vi "16CH Denkovi Manager.vi"(7 "Action":T2=enum."Init", 8 "error in (no error)":errorcluster, 9 "Relay #":i8 min=1 max=8, 10 "Relays In":bool[](array[boolean])=[FALSE, FALSE, FALSE, FALSE, FALSE, FALSE, FALSE, FALSE, FALSE, FALSE, FALSE, FALSE, FALSE, FALSE, FALSE, FALSE]) -> (0 "error out":errorcluster, 2 "Relays Out":bool[](array[boolean]), 4 "Connected":bool)   [LabVIEW 2020]
uses:
  16CH Denkovi Mngr.ctl
  <vilib>/Instr/_visa.llb/VISA Find Search Mode.ctl
  Hardware Globals.vi
panel:
  out "find list 2":string[](array[string])
  out "find list":string[](array[string])
  out "Device Description":string
  out "Pin States":T1
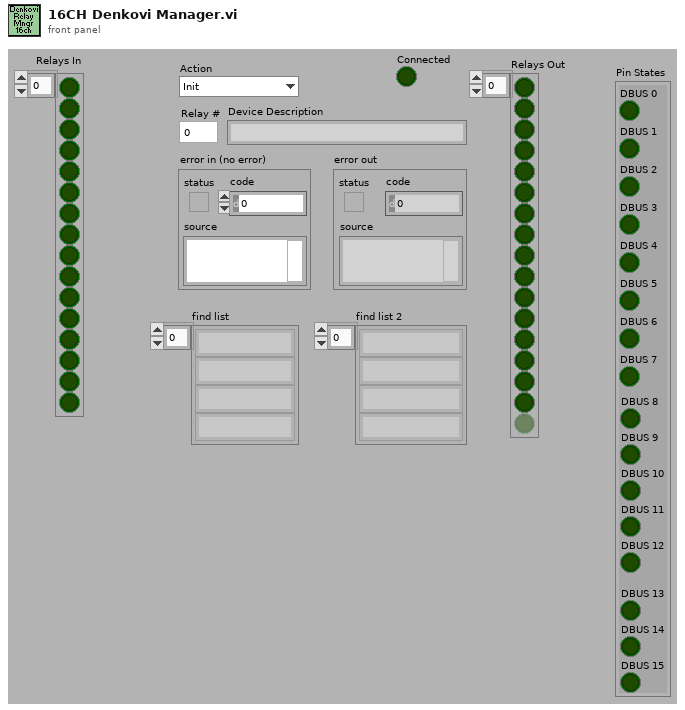
[diagram p1: front panel]
types:
  T1 = cluster{"DBUS 0":bool, "DBUS 1":bool, "DBUS 2":bool, "DBUS 3":bool, "DBUS 4":bool, "DBUS 5":bool, "DBUS 6":bool, "DBUS 7":bool, "DBUS 8":bool, "DBUS 9":bool, "DBUS 10":bool, "DBUS 11":bool, "DBUS 12":bool, "DBUS 13":bool, "DBUS 14":bool, "DBUS 15":bool}
  T2 = typedef "16CH Denkovi Mngr.ctl" = enum16{"Search", "Init", "Set Peristaltic", "Set Pressure", "Set Vacuum", "Pres Vent&Close", "Vac Vent&Close", "Pres ON", "Vac ON", "Set All Relays", "Set One Relay", "Read Relays", "Close"}
  T3 = typedef "VISA Find Search Mode.ctl" = u32
  T4 = cluster{"Boolean array[0]":bool, "Boolean array[1]":bool, "Boolean array[2]":bool, "Boolean array[3]":bool, "Boolean array[4]":bool, "Boolean array[5]":bool, "Boolean array[6]":bool, "Boolean array[7]":bool, "Boolean array[8]":bool, "Boolean array[9]":bool, "Boolean array[10]":bool, "Boolean array[11]":bool, "Boolean array[12]":bool, "Boolean array[13]":bool, "Boolean array[14]":bool, "Boolean array[15]":bool}
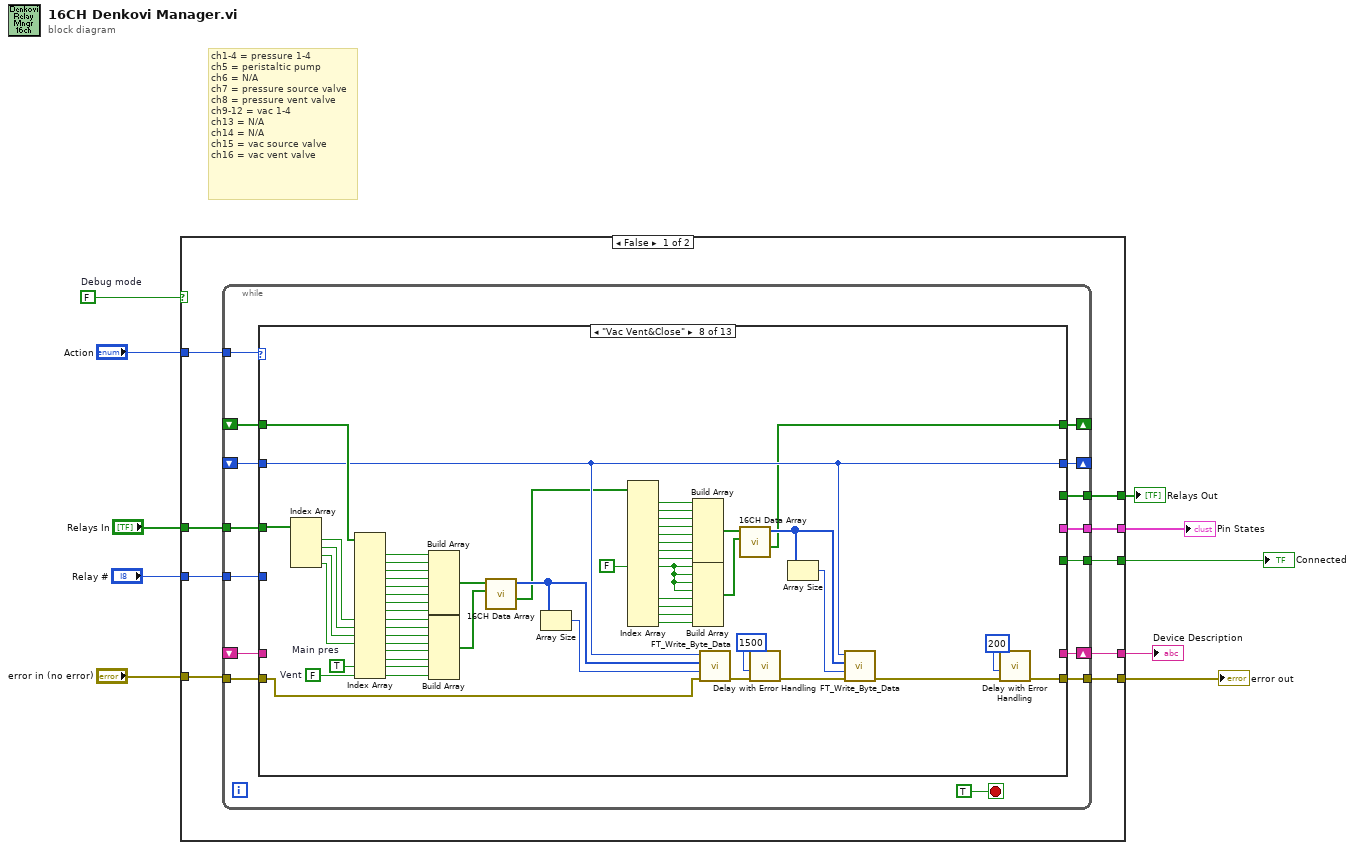
[diagram p0: block diagram]
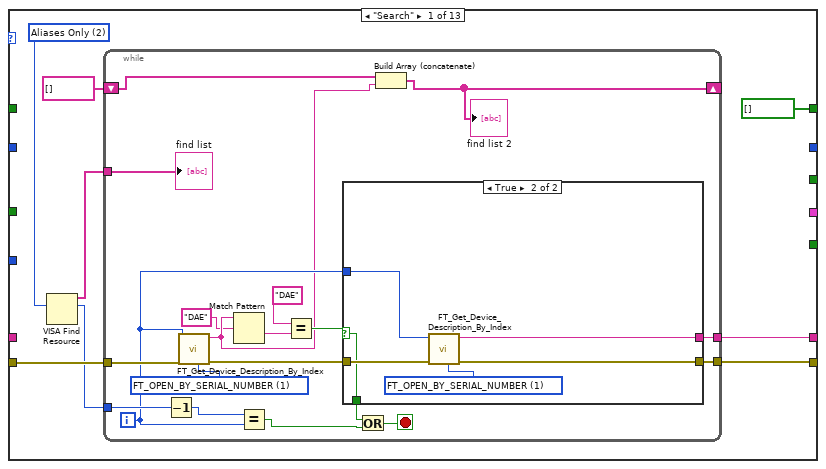
[diagram p2: hidden frame]
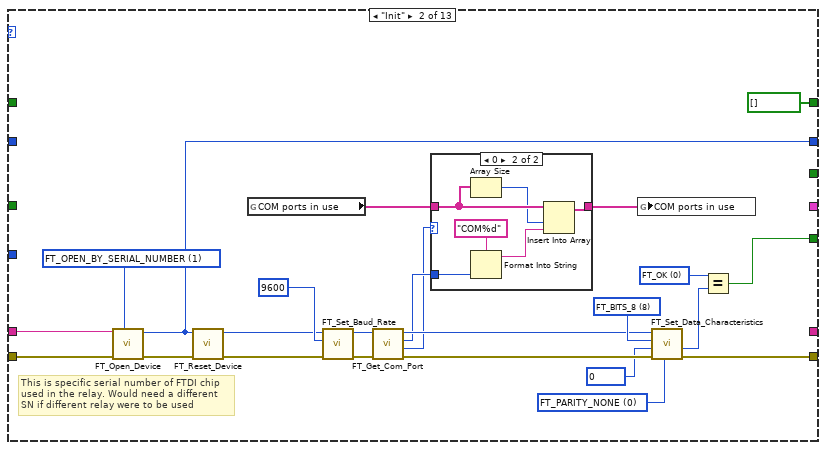
[diagram p4: hidden frame]
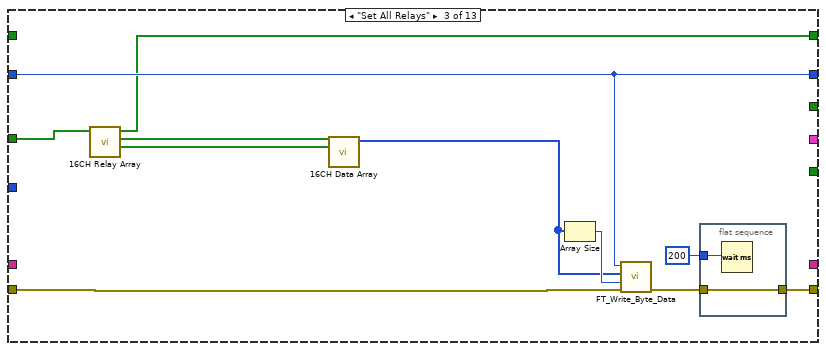
[diagram p6: hidden frame]
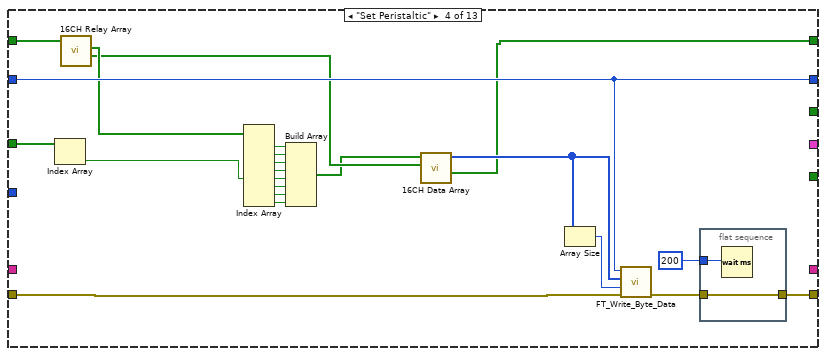
[diagram p7: hidden frame]
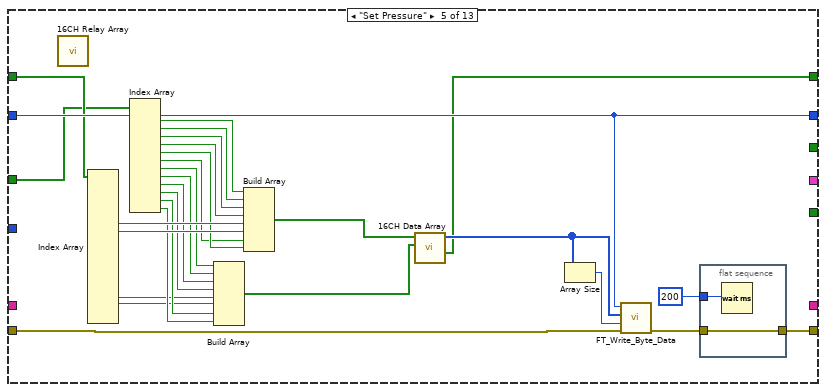
[diagram p8: hidden frame]
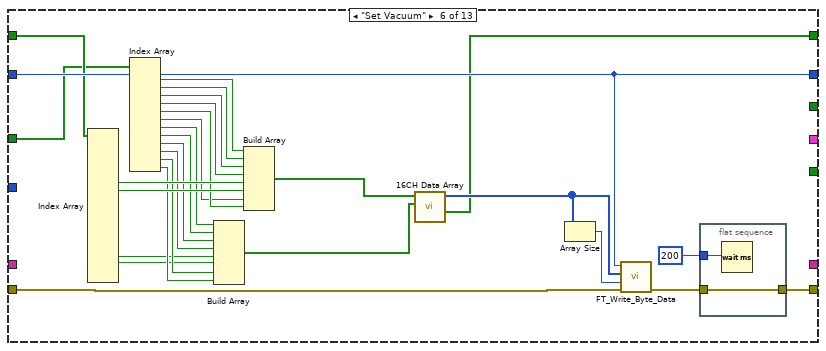
[diagram p9: hidden frame]
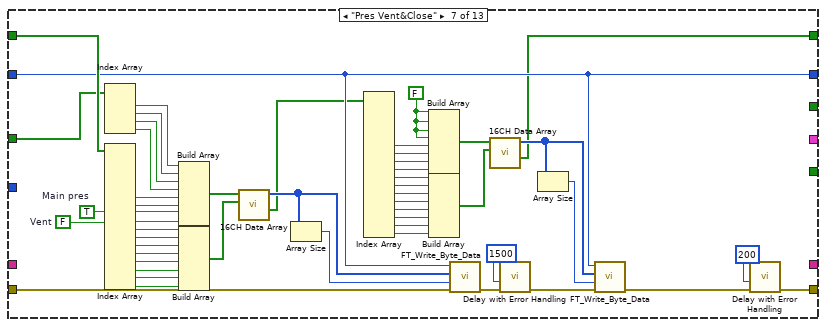
[diagram p10: hidden frame]
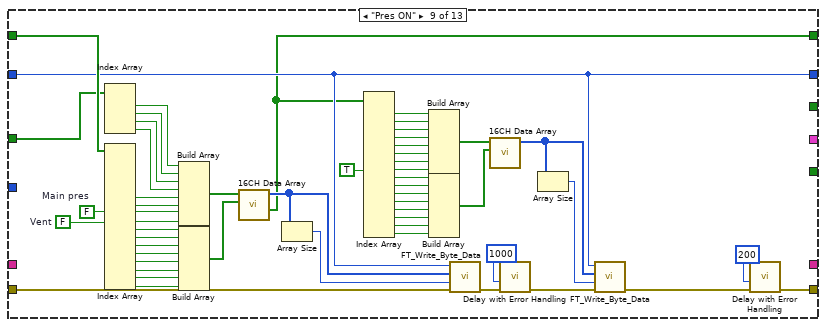
[diagram p11: hidden frame]
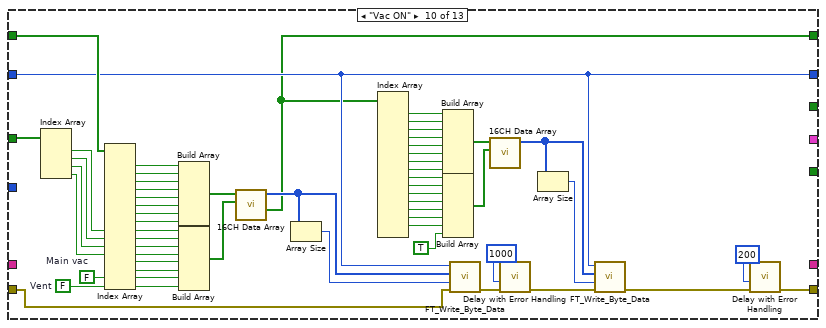
[diagram p12: hidden frame]
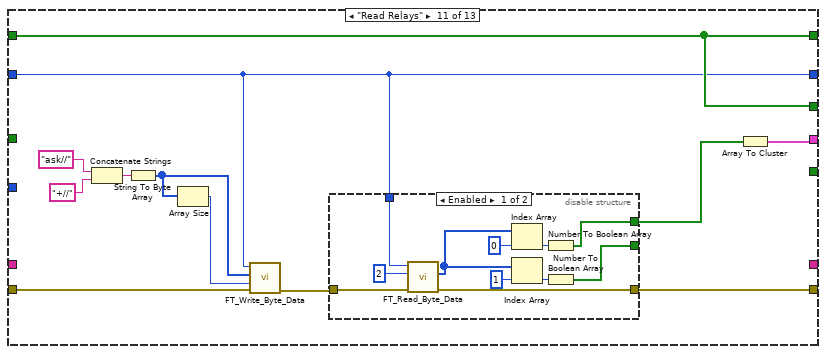
[diagram p13: hidden frame]
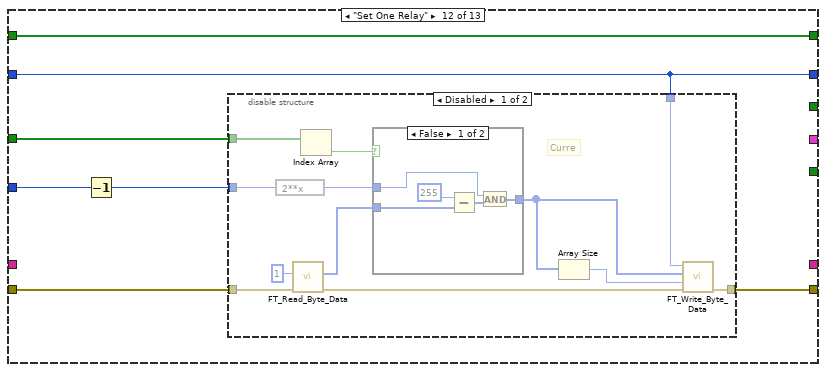
[diagram p15: hidden frame]
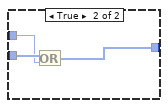
[diagram p16: hidden frame]
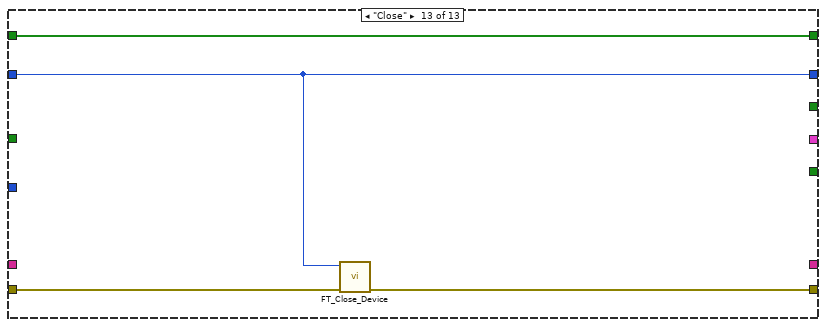
[diagram p18: hidden frame]
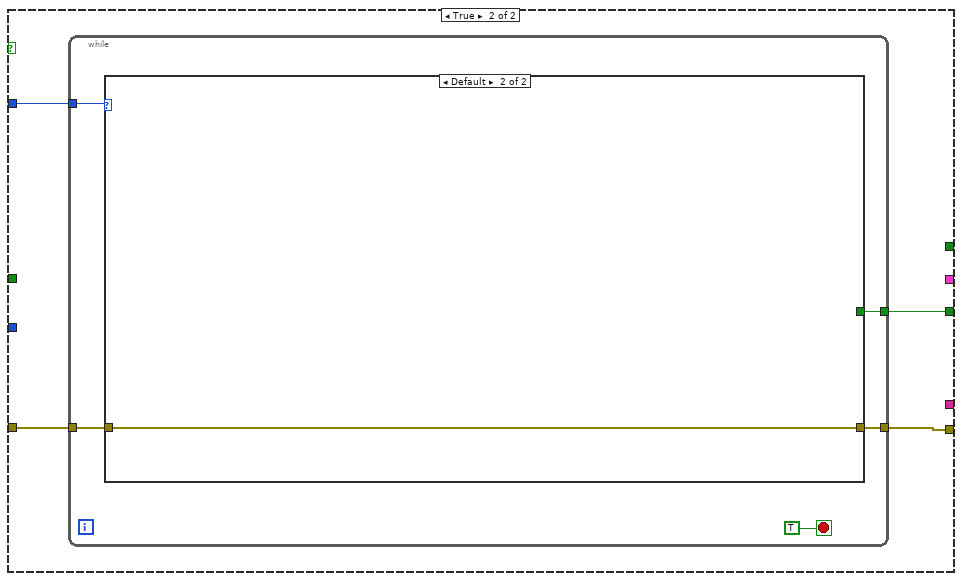
[diagram p19: hidden frame]
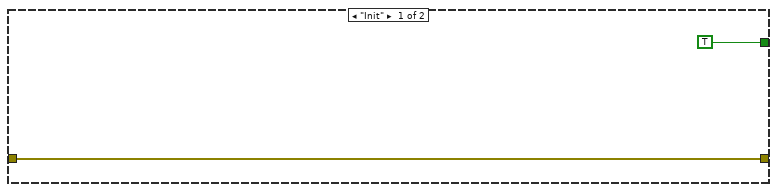
[diagram p20: hidden frame]
diagram:
  w3 = FALSE  # Debug mode
  # "ch1-4 = pressure 1-4\nch5 = peristaltic pump\nch6 = N/A\nch7 = pressure source valve\nch8 = pressure vent valve\nch9-12 = vac 1-4\nch13 = N/A\nch14 = N/A\nch15 = vac source valve\nch16 = vac vent valve"
  n1 = case shown="False" w3 {
    tunnel: [w19 w454] -> w10
    tunnel: "error in (no error)" -> [w18 w453]
    tunnel: "Action" -> [w17 w452]
    tunnel: [w16 w451] -> w7
    tunnel: "Relays In" -> [w15 _]
    tunnel: [w14 _] -> w1
    tunnel: "Relay #" -> [w13 _]
    tunnel: [w12 _] -> w4
    tunnel: [w11 _] -> w2
    frame False {
      n2 = while {
        tunnel: w18 -> [w32]
        tunnel: [w31] -> w19
        tunnel: w17 -> [w33]
        tunnel: [w30] -> w16
        shift-right: [w29] -> _
        shift-left: _ -> [w28]
        tunnel: w15 -> [w27]
        tunnel: [w20] -> w14
        tunnel: w13 -> [w26]
        tunnel: [w25] -> w12
        shift-right: [w24] -> _
        shift-left: _ -> [w23]
        shift-right: [w22] -> w11
        shift-left: _ -> [w21]
        stop <- TRUE stop-if-true
        n3 = case shown="\"Vac Vent&Close\"" w33 {
          tunnel: w32 -> [w42 w82 w106 w128 w158 w188 w242 w291 w342 w393 w404 w422 w450]
          tunnel: [w39 w86 w107 w130 w160 w190 w225 w281 w326 w383 w407 w425 w449] -> w31
          tunnel: [_ w92 _ _ _ _ _ _ _ _ _ _ _] -> w30
          tunnel: [_ w73 w109 w132 w162 w192 w222 w278 w324 w380 w399 w424 w448] -> w29
          tunnel: w28 -> [_ _ w109 w132 w162 w192 w222 w278 w324 w380 w399 w424 w448]
          tunnel: w27 -> [_ _ w104 w124 w154 w184 w238 w256 w338 w359 _ w426 _]
          tunnel: w26 -> [_ _ _ _ _ _ _ _ _ _ _ w423 _]
          tunnel: [_ _ _ _ _ _ _ _ _ _ w406 _ _] -> w25
          tunnel: [bool[] [] ("Relays In") bool[] [] ("Relays In") w100 w113 w136 w166 w196 w245 w299 w350 w406 w420 w447] -> w24
          tunnel: w23 -> [_ _ _ w120 w157 w187 w241 w290 w341 w392 w406 w420 w447]
          tunnel: [w36 _ _ _ _ _ _ _ _ _ _ _ _] -> w22
          tunnel: w21 -> [_ w72 _ _ _ _ _ _ _ _ _ _ _]
          tunnel: [_ _ _ _ _ _ _ _ _ _ w405 _ _] -> w20
          frame "Search" {
            w41 = T3 2 items=["Canonical Names Only"=0, "Aliases Only"=2, "Include Matching Aliases"=3, "Include All Aliases"=4] ("Search Mode")
            n4 = VISA Find Resource(10:w41) -> (2:w40:u32, 3:w37:string[])  [unwired: 2 in, 1 out]
            n5 = while {
              tunnel: w42 -> [w61]
              tunnel: w40 -> [w58]
              tunnel: [w55] -> w39
              tunnel: w37 -> [w53]
              tunnel: [w52] -> w36
              shift-right: [w50] -> _
              shift-left: string[] [] -> [w51]
              i -> [w54]
              stop <- w45 stop-if-true
              w49 = u32 1 items=["FT_OPEN_BY_SERIAL_NUMBER"=1, "FT_OPEN_BY_DESCRIPTION"=2, "FT_OPEN_BY_LOCATION"=4] ("Flags")
              n6 = Decrement(x=w58) -> (x-1=w57:u32)
              n7 = call "FT_Get_Device_Description_By_Index.vi"("Flags"=w49, "error in (no error)"=w61, "Device Index"=w54) -> ("error out"=w59:errorcluster, "Device Description"=w44:string)  [unwired: 6 in, 1 out]
              n8 = Match Pattern(string=w44, regular expression="DAE" ("string")) -> (match substring=w48:string)  [unwired: 1 in, 3 out]
              n9 = Equal?(x=w57, y=w54) -> (x = y?=w47:bool)
              n10 = Equal?(x="DAE", y=w48) -> (x = y?=w56:bool)
              n11 = case shown="True" w56 {
                selector: w56 -> [_ w64]
                tunnel: w59 -> [w62 w68]
                tunnel: [w62 w66] -> w55
                tunnel: w54 -> [_ w67]
                tunnel: [_ w65] -> w52
                tunnel: [_ w64] -> w46
                frame False {
                }
                frame True {
                  w63 = u32 1 items=["FT_OPEN_BY_SERIAL_NUMBER"=1, "FT_OPEN_BY_DESCRIPTION"=2, "FT_OPEN_BY_LOCATION"=4] ("Flags")
                  n12 = call "FT_Get_Device_Description_By_Index.vi"("Flags"=w63, "error in (no error)"=w68, "Device Index"=w67) -> ("error out"=w66:errorcluster, "Device Description"=w65:string)  [unwired: 6 in, 1 out]
                }
              }
              n13 = Or(x=w46, y=w47) -> (x .or. y?=w45:bool)
              n14 = Build Array (concatenate)(w51, w44) -> (w50:string[])
              "find list 2" <- w50
              "find list" <- w53
            }
          }
          frame "Init" {
            w71 = u8 0 items=["FT_STOP_BITS_1"=1, "FT_STOP_BITS_2"=2] ("Stop Bits")
            w83 = u32 1 items=["FT_OPEN_BY_SERIAL_NUMBER"=1, "FT_OPEN_BY_DESCRIPTION"=2, "FT_OPEN_BY_LOCATION"=4] ("Flags")
            w89 = u8 0 items=["FT_PARITY_NONE", "FT_PARITY_ODD", "FT_PARITY_EVEN", "FT_PARITY_MARK", "FT_PARITY_SPACE"] ("Parity")
            w88 = u8 8 items=["FT_BITS_7"=7, "FT_BITS_8"=8] ("Word Length")
            w91 = u32 0 items=["FT_OK", "FT_INVALID_HANDLE", "FT_DEVICE_NOT_FOUND", "FT_DEVICE_NOT_OPENED", "FT_IO_ERROR", "FT_INSUFFICIENT_RESOURCES", "FT_INVALID_PARAMETER", "FT_INVALID_BAUD_RATE", "FT_DEVICE_NOT_OPENED_FOR_ERASE", "FT_DEVICE_NOT_OPENED_FOR_WRITE", "FT_FAILED_TO_WRITE_DEVICE", "FT_EEPROM_READ_FAILED", "FT_EEPROM_WRITE_FAILED", "FT_EEPROM_ERASE_FAILED", "FT_EEPROM_NOT_PRESENT", "FT_EEPROM_NOT_PROGRAMMED", "FT_INVALID_ARGS", "FT_NOT_SUPPORTED", "FT_OTHER_ERROR"] ("FT_Status")
            # "This is specific serial number of FTDI chip\nused in the relay. Would need a different\nSN if different relay were to be used"
            n15 = call "FT_Open_Device.vi"("Flags"=w83, "error in (no error)"=w82, "Device Description"=w72) -> ("error out"=w85:errorcluster, "Handle"=w73:u64)  [unwired: 6 in, 1 out]
            n16 = call "FT_Reset_Device.vi"("error in (no error)"=w85, "Handle In"=w73) -> ("error out"=w69:errorcluster, "Handle Out"=w70:u64)  [unwired: 7 in, 1 out]
            n17 = global read "Hardware Globals.vi" "COM ports in use"() -> (w76:string[])
            n18 = call "FT_Set_Baud_Rate.vi"("error in (no error)"=w69, "Baud Rate"=9600, "Handle  In"=w70) -> ("error out"=w81:errorcluster, "Handle Out"=w80:u64)  [unwired: 6 in, 1 out]
            n19 = call "FT_Get_Com_Port.vi"("error in (no error)"=w81, "Handle In"=w80) -> ("error out"=w78:errorcluster, "FT_Status"=w74:u32, "ComPortNumber"=w77:i32, "Handle Out"=w79:u64)  [unwired: 6 in]
            n20 = case shown="0" w74 {
              tunnel: w77 -> [_ w99]
              tunnel: w76 -> [w93 w97]
              tunnel: [w93 w94] -> w75
              frame Default {
              }
              frame 0 {
                n21 = Array Size(array=w97) -> (size(s)=w96:i32)
                n22 = Format Into String(format string="COM%d", w99) -> (resulting string=w95:string)  [unwired: 2 in, 1 out]
                n23 = Insert Into Array(array=w97, index=w96, new element=w95) -> (w94:string[])
              }
            }
            n24 = global write "Hardware Globals.vi" "COM ports in use"(w75) -> ()
            n25 = call "FT_Set_Data_Characteristics.vi"("Parity"=w89, "error in"=w78, "Stop Bits"=w71, "Word Length"=w88, "Handle In"=w79) -> ("error out"=w86:errorcluster, "FT_Status"=w87:u32)  [unwired: 4 in, 1 out]
            n26 = Equal?(x=w91, y=w87) -> (x = y?=w92:bool)
          }
          frame "Set All Relays" {
            n27 = call "16CH Relay Array.vi"("Relays In"=w104) -> ("Relays 9-16"=w102:bool[], "Relays 1-8"=w103:bool[], "Relays 1-16"=w100:bool[])  [unwired: 8 in]
            n28 = call "16CH Data Array.vi"("Relays 9-16"=w102, "Relays 1-8"=w103) -> ("unsigned byte array"=w105:u8[])  [unwired: 8 in, 1 out]
            n29 = Array Size(array=w105) -> (size(s)=w110:i32)
            n30 = call "FT_Write_Byte_Data.vi"("error in (no error)"=w106, "Bytes To Write"=w110, "Buffer"=w105, "Handle"=w109) -> ("error out"=w108:errorcluster)  [unwired: 4 in, 3 out]
            n31 = flat-sequence {
              tunnel: w108 -> [w112]
              tunnel: [w112] -> w107
              tunnel: u32 200 ("Delay (ms)") -> [w111]
              frame #0 {
                n32 = Wait (ms)(milliseconds to wait=w111) -> ()  [unwired: 1 out]
              }
            }
          }
          frame "Set Peristaltic" {
            n33 = Index Array(array=w124) -> (element=w114:bool)  [unwired: 1 in]
            n34 = call "16CH Relay Array.vi"("Relays In"=w120) -> ("Relays 9-16"=w118:bool[], "Relays 1-8"=w119:bool[])  [unwired: 8 in, 1 out]
            n35 = Index Array(array=w119) -> (element #1=w127:bool, element #2=w126:bool, element #3=w125:bool, element #4=w115:bool, element #6=w121:bool, element #7=w122:bool, element #8=w123:bool)  [unwired: 8 in, 1 out]
            n36 = Build Array(w127, w126, w125, w115, w114, w121, w122, w123) -> (w117:bool[])
            n37 = call "16CH Data Array.vi"("Relays 9-16"=w118, "Relays 1-8"=w117) -> ("Relays 1-16"=w113:bool[], "unsigned byte array"=w116:u8[])  [unwired: 8 in]
            n38 = Array Size(array=w116) -> (size(s)=w133:i32)
            n39 = call "FT_Write_Byte_Data.vi"("error in (no error)"=w128, "Bytes To Write"=w133, "Buffer"=w116, "Handle"=w132) -> ("error out"=w131:errorcluster)  [unwired: 4 in, 3 out]
            n40 = flat-sequence {
              tunnel: w131 -> [w135]
              tunnel: [w135] -> w130
              tunnel: u32 200 ("Delay (ms)") -> [w134]
              frame #0 {
                n41 = Wait (ms)(milliseconds to wait=w134) -> ()  [unwired: 1 out]
              }
            }
          }
          frame "Set Pressure" {
            n42 = call "16CH Relay Array.vi"() -> ()  [unwired: 9 in, 3 out]
            n43 = Index Array(array=w157) -> (element #5=w155:bool, element #6=w156:bool, element #14=w140:bool, element #15=w141:bool)  [unwired: 17 in, 13 out]
            n44 = Index Array(array=w154) -> (element #1=w153:bool, element #2=w152:bool, element #3=w151:bool, element #4=w150:bool, element #5=w149:bool, element #6=w148:bool, element #7=w142:bool, element #8=w143:bool, element #9=w144:bool, element #10=w145:bool, element #11=w146:bool, element #12=w147:bool)  [unwired: 12 in]
            n45 = Build Array(w142, w143, w144, w145, w140, w141, w146, w147) -> (w137:bool[])
            n46 = Build Array(w153, w152, w151, w150, w155, w156, w148, w149) -> (w138:bool[])
            n47 = call "16CH Data Array.vi"("Relays 9-16"=w137, "Relays 1-8"=w138) -> ("Relays 1-16"=w136:bool[], "unsigned byte array"=w139:u8[])  [unwired: 8 in]
            n48 = Array Size(array=w139) -> (size(s)=w163:i32)
            n49 = call "FT_Write_Byte_Data.vi"("error in (no error)"=w158, "Bytes To Write"=w163, "Buffer"=w139, "Handle"=w162) -> ("error out"=w161:errorcluster)  [unwired: 4 in, 3 out]
            n50 = flat-sequence {
              tunnel: w161 -> [w165]
              tunnel: [w165] -> w160
              tunnel: u32 200 ("Delay (ms)") -> [w164]
              frame #0 {
                n51 = Wait (ms)(milliseconds to wait=w164) -> ()  [unwired: 1 out]
              }
            }
          }
          frame "Set Vacuum" {
            n52 = Index Array(array=w187) -> (element #5=w185:bool, element #6=w186:bool, element #14=w170:bool, element #15=w171:bool)  [unwired: 17 in, 13 out]
            n53 = Index Array(array=w184) -> (element #1=w183:bool, element #2=w182:bool, element #3=w181:bool, element #4=w180:bool, element #5=w179:bool, element #6=w178:bool, element #7=w172:bool, element #8=w173:bool, element #9=w174:bool, element #10=w175:bool, element #11=w176:bool, element #12=w177:bool)  [unwired: 12 in]
            n54 = Build Array(w172, w173, w174, w175, w170, w171, w176, w177) -> (w167:bool[])
            n55 = Build Array(w183, w182, w181, w180, w185, w186, w178, w179) -> (w168:bool[])
            n56 = call "16CH Data Array.vi"("Relays 9-16"=w167, "Relays 1-8"=w168) -> ("Relays 1-16"=w166:bool[], "unsigned byte array"=w169:u8[])  [unwired: 8 in]
            n57 = Array Size(array=w169) -> (size(s)=w193:i32)
            n58 = call "FT_Write_Byte_Data.vi"("error in (no error)"=w188, "Bytes To Write"=w193, "Buffer"=w169, "Handle"=w192) -> ("error out"=w191:errorcluster)  [unwired: 4 in, 3 out]
            n59 = flat-sequence {
              tunnel: w191 -> [w195]
              tunnel: [w195] -> w190
              tunnel: u32 200 ("Delay (ms)") -> [w194]
              frame #0 {
                n60 = Wait (ms)(milliseconds to wait=w194) -> ()  [unwired: 1 out]
              }
            }
          }
          frame "Pres Vent&Close" {
            w221 = TRUE  # Main pres
            w227 = FALSE ("element")
            w233 = FALSE  # Vent
            n61 = Index Array(array=w238) -> (element #1=w237:bool, element #2=w236:bool, element #3=w235:bool, element #4=w234:bool)  [unwired: 4 in]
            n62 = Index Array(array=w241) -> (element #5=w239:bool, element #6=w240:bool, element #9=w217:bool, element #10=w216:bool, element #11=w215:bool, element #12=w214:bool, element #13=w213:bool, element #14=w212:bool, element #15=w211:bool, element #16=w210:bool)  [unwired: 16 in, 6 out]
            n63 = Build Array(w237, w236, w235, w234, w239, w240, w221, w233) -> (w219:bool[])
            n64 = Build Array(w217, w216, w215, w214, w213, w212, w211, w210) -> (w209:bool[])
            n65 = call "16CH Data Array.vi"("Relays 9-16"=w209, "Relays 1-8"=w219) -> ("Relays 1-16"=w197:bool[], "unsigned byte array"=w218:u8[])  [unwired: 8 in]
            n66 = Array Size(array=w218) -> (size(s)=w244:i32)
            n67 = Index Array(array=w197) -> (element #5=w230:bool, element #6=w229:bool, element #7=w228:bool, element #8=w223:bool, element #9=w208:bool, element #10=w207:bool, element #11=w206:bool, element #12=w205:bool, element #13=w204:bool, element #14=w203:bool, element #15=w202:bool, element #16=w201:bool)  [unwired: 16 in, 4 out]
            n68 = Build Array(w227, w227, w227, w227, w230, w229, w228, w223) -> (w200:bool[])
            n69 = Build Array(w208, w207, w206, w205, w204, w203, w202, w201) -> (w198:bool[])
            n70 = call "FT_Write_Byte_Data.vi"("error in (no error)"=w242, "Bytes To Write"=w244, "Buffer"=w218, "Handle"=w222) -> ("error out"=w243:errorcluster)  [unwired: 4 in, 3 out]
            n71 = call "16CH Data Array.vi"("Relays 9-16"=w198, "Relays 1-8"=w200) -> ("Relays 1-16"=w196:bool[], "unsigned byte array"=w199:u8[])  [unwired: 8 in]
            n72 = call "Delay with Error Handling.vi"("error in (no error)"=w243, "Delay (ms)"=u32 1500) -> ("error out"=w224:errorcluster)  [unwired: 9 in]
            n73 = Array Size(array=w199) -> (size(s)=w231:i32)
            n74 = call "FT_Write_Byte_Data.vi"("error in (no error)"=w224, "Bytes To Write"=w231, "Buffer"=w199, "Handle"=w222) -> ("error out"=w220:errorcluster)  [unwired: 4 in, 3 out]
            n75 = call "Delay with Error Handling.vi"("error in (no error)"=w220, "Delay (ms)"=u32 200) -> ("error out"=w225:errorcluster)  [unwired: 9 in]
          }
          frame "Vac Vent&Close" {
            w264 = TRUE  # Main pres
            w247 = FALSE ("element")
            w265 = FALSE  # Vent
            n76 = Index Array(array=w256) -> (element #1=w255:bool, element #2=w254:bool, element #3=w253:bool, element #4=w252:bool)  [unwired: 4 in]
            n77 = Index Array(array=w290) -> (element #1=w257:bool, element #2=w258:bool, element #3=w259:bool, element #4=w260:bool, element #5=w288:bool, element #6=w289:bool, element #7=w261:bool, element #8=w262:bool, element #13=w274:bool, element #14=w263:bool)  [unwired: 16 in, 6 out]
            n78 = Build Array(w257, w258, w259, w260, w288, w289, w261, w262) -> (w276:bool[])
            n79 = Build Array(w255, w254, w253, w252, w274, w263, w264, w265) -> (w273:bool[])
            n80 = call "16CH Data Array.vi"("Relays 9-16"=w273, "Relays 1-8"=w276) -> ("Relays 1-16"=w246:bool[], "unsigned byte array"=w275:u8[])  [unwired: 8 in]
            n81 = Array Size(array=w275) -> (size(s)=w293:i32)
            n82 = Index Array(array=w246) -> (element #1=w248:bool, element #2=w249:bool, element #3=w250:bool, element #4=w251:bool, element #5=w285:bool, element #6=w284:bool, element #7=w283:bool, element #8=w279:bool, element #13=w272:bool, element #14=w271:bool, element #15=w270:bool, element #16=w269:bool)  [unwired: 16 in, 4 out]
            n83 = Build Array(w248, w249, w250, w251, w285, w284, w283, w279) -> (w268:bool[])
            n84 = Build Array(w247, w247, w247, w247, w272, w271, w270, w269) -> (w266:bool[])
            n85 = call "FT_Write_Byte_Data.vi"("error in (no error)"=w291, "Bytes To Write"=w293, "Buffer"=w275, "Handle"=w278) -> ("error out"=w292:errorcluster)  [unwired: 4 in, 3 out]
            n86 = call "16CH Data Array.vi"("Relays 9-16"=w266, "Relays 1-8"=w268) -> ("Relays 1-16"=w245:bool[], "unsigned byte array"=w267:u8[])  [unwired: 8 in]
            n87 = call "Delay with Error Handling.vi"("error in (no error)"=w292, "Delay (ms)"=u32 1500) -> ("error out"=w280:errorcluster)  [unwired: 9 in]
            n88 = Array Size(array=w267) -> (size(s)=w286:i32)
            n89 = call "FT_Write_Byte_Data.vi"("error in (no error)"=w280, "Bytes To Write"=w286, "Buffer"=w267, "Handle"=w278) -> ("error out"=w277:errorcluster)  [unwired: 4 in, 3 out]
            n90 = call "Delay with Error Handling.vi"("error in (no error)"=w277, "Delay (ms)"=u32 200) -> ("error out"=w281:errorcluster)  [unwired: 9 in]
          }
          frame "Pres ON" {
            w323 = FALSE  # Main pres
            w333 = FALSE  # Vent
            n91 = Index Array(array=w338) -> (element #1=w337:bool, element #2=w336:bool, element #3=w335:bool, element #4=w334:bool)  [unwired: 4 in]
            n92 = Index Array(array=w341) -> (element #5=w339:bool, element #6=w340:bool, element #9=w319:bool, element #10=w318:bool, element #11=w317:bool, element #12=w316:bool, element #13=w315:bool, element #14=w314:bool, element #15=w313:bool, element #16=w312:bool)  [unwired: 16 in, 6 out]
            n93 = Build Array(w337, w336, w335, w334, w339, w340, w323, w333) -> (w321:bool[])
            n94 = Build Array(w319, w318, w317, w316, w315, w314, w313, w312) -> (w311:bool[])
            n95 = call "16CH Data Array.vi"("Relays 9-16"=w311, "Relays 1-8"=w321) -> ("Relays 1-16"=w299:bool[], "unsigned byte array"=w320:u8[])  [unwired: 8 in]
            n96 = Array Size(array=w320) -> (size(s)=w344:i32)
            n97 = Index Array(array=w299) -> (element #1=w298:bool, element #2=w297:bool, element #3=w296:bool, element #4=w295:bool, element #5=w330:bool, element #6=w329:bool, element #7=w328:bool, element #9=w310:bool, element #10=w309:bool, element #11=w308:bool, element #12=w307:bool, element #13=w306:bool, element #14=w305:bool, element #15=w304:bool, element #16=w303:bool)  [unwired: 16 in, 1 out]
            n98 = Build Array(w298, w297, w296, w295, w330, w329, w328, TRUE ("element")) -> (w302:bool[])
            n99 = Build Array(w310, w309, w308, w307, w306, w305, w304, w303) -> (w300:bool[])
            n100 = call "FT_Write_Byte_Data.vi"("error in (no error)"=w342, "Bytes To Write"=w344, "Buffer"=w320, "Handle"=w324) -> ("error out"=w343:errorcluster)  [unwired: 4 in, 3 out]
            n101 = call "16CH Data Array.vi"("Relays 9-16"=w300, "Relays 1-8"=w302) -> ("unsigned byte array"=w301:u8[])  [unwired: 8 in, 1 out]
            n102 = call "Delay with Error Handling.vi"("error in (no error)"=w343, "Delay (ms)"=u32 1000) -> ("error out"=w325:errorcluster)  [unwired: 9 in]
            n103 = Array Size(array=w301) -> (size(s)=w331:i32)
            n104 = call "FT_Write_Byte_Data.vi"("error in (no error)"=w325, "Bytes To Write"=w331, "Buffer"=w301, "Handle"=w324) -> ("error out"=w322:errorcluster)  [unwired: 4 in, 3 out]
            n105 = call "Delay with Error Handling.vi"("error in (no error)"=w322, "Delay (ms)"=u32 200) -> ("error out"=w326:errorcluster)  [unwired: 9 in]
          }
          frame "Vac ON" {
            w367 = FALSE  # Main vac
            w368 = FALSE  # Vent
            n106 = Index Array(array=w359) -> (element #1=w358:bool, element #2=w357:bool, element #3=w356:bool, element #4=w355:bool)  [unwired: 4 in]
            n107 = Index Array(array=w392) -> (element #1=w360:bool, element #2=w361:bool, element #3=w362:bool, element #4=w363:bool, element #5=w390:bool, element #6=w391:bool, element #7=w364:bool, element #8=w365:bool, element #13=w376:bool, element #14=w366:bool)  [unwired: 16 in, 6 out]
            n108 = Build Array(w360, w361, w362, w363, w390, w391, w364, w365) -> (w378:bool[])
            n109 = Build Array(w358, w357, w356, w355, w376, w366, w367, w368) -> (w375:bool[])
            n110 = call "16CH Data Array.vi"("Relays 9-16"=w375, "Relays 1-8"=w378) -> ("Relays 1-16"=w350:bool[], "unsigned byte array"=w377:u8[])  [unwired: 8 in]
            n111 = Array Size(array=w377) -> (size(s)=w395:i32)
            n112 = Index Array(array=w350) -> (element #1=w351:bool, element #2=w352:bool, element #3=w353:bool, element #4=w354:bool, element #5=w387:bool, element #6=w386:bool, element #7=w385:bool, element #8=w381:bool, element #9=w349:bool, element #10=w348:bool, element #11=w347:bool, element #12=w346:bool, element #13=w374:bool, element #14=w373:bool, element #15=w372:bool)  [unwired: 16 in, 1 out]
            n113 = Build Array(w351, w352, w353, w354, w387, w386, w385, w381) -> (w371:bool[])
            n114 = Build Array(w349, w348, w347, w346, w374, w373, w372, TRUE ("element")) -> (w369:bool[])
            n115 = call "FT_Write_Byte_Data.vi"("error in (no error)"=w393, "Bytes To Write"=w395, "Buffer"=w377, "Handle"=w380) -> ("error out"=w394:errorcluster)  [unwired: 4 in, 3 out]
            n116 = call "16CH Data Array.vi"("Relays 9-16"=w369, "Relays 1-8"=w371) -> ("unsigned byte array"=w370:u8[])  [unwired: 8 in, 1 out]
            n117 = call "Delay with Error Handling.vi"("error in (no error)"=w394, "Delay (ms)"=u32 1000) -> ("error out"=w382:errorcluster)  [unwired: 9 in]
            n118 = Array Size(array=w370) -> (size(s)=w388:i32)
            n119 = call "FT_Write_Byte_Data.vi"("error in (no error)"=w382, "Bytes To Write"=w388, "Buffer"=w370, "Handle"=w380) -> ("error out"=w379:errorcluster)  [unwired: 4 in, 3 out]
            n120 = call "Delay with Error Handling.vi"("error in (no error)"=w379, "Delay (ms)"=u32 200) -> ("error out"=w383:errorcluster)  [unwired: 9 in]
          }
          frame "Read Relays" {
            n121 = Concatenate Strings("ask//" ("string"), "+//" ("string")) -> (w400:string)
            n122 = String To Byte Array(string=w400) -> (unsigned byte array=w398:u8[])
            n123 = Array Size(array=w398) -> (size(s)=w397:i32)
            n124 = call "FT_Write_Byte_Data.vi"("error in (no error)"=w404, "Bytes To Write"=w397, "Buffer"=w398, "Handle"=w399) -> ("error out"=w403:errorcluster)  [unwired: 4 in, 3 out]
            n125 = disable-structure shown="Enabled" {
              disable-tunnel: [w418 w419] -> w407
              disable-tunnel: w403 -> [w417 w419]
              disable-tunnel: w399 -> [w416 _]
              disable-tunnel: [w409 _] -> w396
              disable-tunnel: [w408 _] -> _
              frame Enabled {
                n126 = call "FT_Read_Byte_Data.vi"("error in (no error)"=w417, "Bytes To Read"=2, "Handle In"=w416) -> ("error out"=w418:errorcluster, "Read Data"=w410:u8[])  [unwired: 4 in, 3 out]
                n127 = Index Array(array=w410, index=0) -> (element=w414:u8)
                n128 = Index Array(array=w410, index=1) -> (element=w412:u8)
                n129 = Number To Boolean Array(number=w414) -> (Boolean array=w409:bool[])
                n130 = Number To Boolean Array(number=w412) -> (Boolean array=w408:bool[])
              }
              frame Disabled {
              }
            }
            n131 = Array To Cluster(array=w396) -> (cluster=w405:T4)
          }
          frame "Set One Relay" {
            n132 = Decrement(x=w423) -> (x-1=w421:i8)
            n133 = disable-structure shown="Disabled" {
              disable-tunnel: w426 -> [w437 _]
              disable-tunnel: [w436 _] -> w425
              disable-tunnel: w424 -> [w435 _]
              disable-tunnel: w422 -> [w432 _]
              disable-tunnel: w421 -> [w431 _]
              frame Disabled {
                # "Curre"
                n134 = expression code="2**x"(w431) -> (w428:i8)
                n135 = call "FT_Read_Byte_Data.vi"("error in (no error)"=w432, "Bytes To Read"=u32 1) -> ("error out"=w433:errorcluster, "Read Data"=w429:u8[])  [unwired: 5 in, 3 out]
                n136 = Index Array(array=w437) -> (element=w427:bool)  [unwired: 1 in]
                n137 = case shown="False" w427 {
                  tunnel: [w441 w444] -> w434
                  tunnel: w429 -> [w440 w446]
                  tunnel: w428 -> [w439 w445]
                  frame False {
                    n138 = Subtract(x=255, y=w440) -> (x-y=w443:i32[])
                    n139 = And(x=w439, y=w443) -> (x .and. y?=w441:i32[])
                  }
                  frame True {
                    n140 = Or(x=w446, y=w445) -> (x .or. y?=w444:u8[])
                  }
                }
                n141 = Array Size(array=w434) -> (size(s)=w438:i32)
                n142 = call "FT_Write_Byte_Data.vi"("error in (no error)"=w433, "Bytes To Write"=w438, "Buffer"=w434, "Handle"=w435) -> ("error out"=w436:errorcluster)  [unwired: 4 in, 3 out]
              }
              frame Enabled {
              }
            }
          }
          frame "Close" {
            n143 = call "FT_Close_Device.vi"("error in (no error)"=w450, "Handle In"=w448) -> ("error out"=w449:errorcluster)  [unwired: 7 in, 2 out]
          }
        }
      }
    }
    frame True {
      n144 = while {
        tunnel: w453 -> [w457]
        tunnel: [w456] -> w454
        tunnel: w452 -> [w458]
        tunnel: [w455] -> w451
        stop <- TRUE stop-if-true
        n145 = case shown="Default" w458 {
          tunnel: w457 -> [w460 w462]
          tunnel: [w460 w462] -> w456
          tunnel: [TRUE _] -> w455
          frame "Init" {
          }
          frame Default {
          }
        }
      }
    }
  }
  "error out" <- w10
  "Connected" <- w7
  "Pin States" <- w1
  "Relays Out" <- w4
  "Device Description" <- w2
